vi "Expand FIFO Type Def.vi"(8 "error in (no error)":errorcluster, 11 "Cluster in":refnum<vi>) -> (0 "error out":errorcluster, 2 "Clsuter Item":refnum<vi>, 3 "Cluster out":refnum<vi>)   [LabVIEW 2014, in "Initialization and IO Node Scripting.lvlib"]
uses:
  Initialization and IO Node Scripting.lvlib
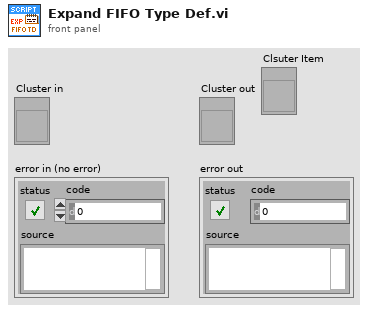
[diagram p1: front panel]
types:
  T1 = typedef "LVPositionTypeDef.ctl" = cluster{"Left":i32, "Top":i32}
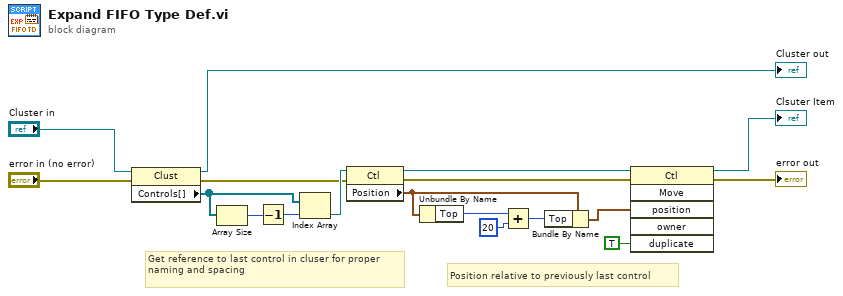
[diagram p0: block diagram]
diagram:
  # "Position relative to previously last control"
  # "Get reference to last control in cluser for proper naming and spacing"
  n1 = property class="Clust"(reference="Cluster in", error in="error in (no error)") -> (reference out=→"Cluster out":refnum<vi>, error out=w5:errorcluster, "Controls[]"=w4:refnum<vi>[])
  n2 = Array Size(array=w4) -> (size(s)=w14:i32)
  n3 = Decrement(x=w14) -> (x-1=w3:i32)
  n4 = Index Array(array=w4, index=w3) -> (element=w10:refnum<vi>)
  n5 = property class="Ctl"(reference=w10, error in=w5) -> (reference out=w11:refnum<vi>, error out=w12:errorcluster, "Position"=w8:T1)
  n6 = Unbundle By Name(w8) -> ("Top"=w7:i32)
  n7 = Add(x=w7, y=20) -> (x+y=w6:i32)
  n8 = Bundle By Name(cluster=w8, "Top"=w6) -> (w9:T1)
  n9 = invoke class="Ctl" method="Move"(reference=w11, error in=w12, "position"=w9, "duplicate"=TRUE ("Duplicate? (F)")) -> (reference out=→"Clsuter Item":refnum<vi>, error out=→"error out":errorcluster)  [unwired: 2 in, 4 out]
